vi "Mathematical_operations.vi"() -> ()   [LabVIEW 2019]
doc: "A vi which has the options to Add, Subtract, Multiply, Divide, Minimum and Maximum of two numbers namely A and B and to find the square and square root of A"
panel:
  in  "stop":bool
  in  "Enum":T1(ring)
  out "Result":dbl
  in  "B":dbl
  in  "A":dbl
  # "Mathematical Operations"
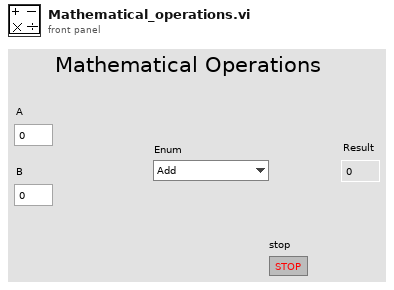
[diagram p1: front panel]
types:
  T1 = enum16{"Add", "Subtract", "Multiply", "Divide", "Square of A", "Square Root of A", "Average", "Minimum", "Maximum"}
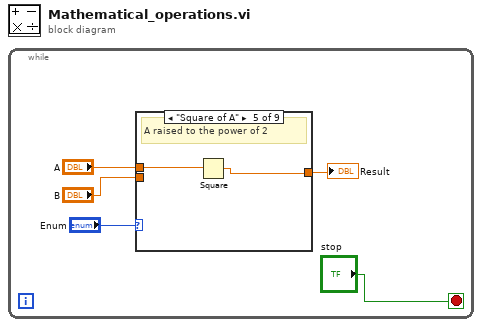
[diagram p0: block diagram]
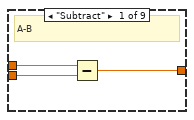
[diagram p2: hidden frame]
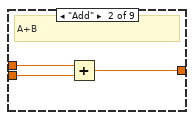
[diagram p3: hidden frame]
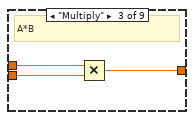
[diagram p4: hidden frame]
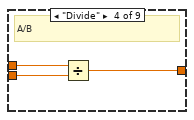
[diagram p5: hidden frame]
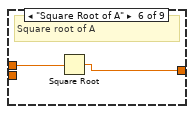
[diagram p6: hidden frame]
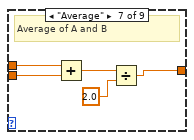
[diagram p7: hidden frame]
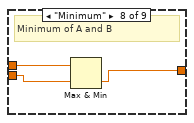
[diagram p8: hidden frame]
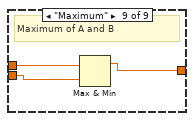
[diagram p9: hidden frame]
diagram:
  n1 = while {
    stop <- "stop" stop-if-true
    n2 = case shown="\"Square of A\"" "Enum" {
      tunnel: "A" -> [w8 w11 w14 w17 w19 w21 w26 w29 w32]
      tunnel: "B" -> [w7 w10 w13 w16 _ _ w25 w28 w31]
      tunnel: [w6 w9 w12 w15 w18 w20 w22 w27 w30] -> w2
      frame "Subtract" {
        # "A-B"
        n3 = Subtract(x=w8, y=w7) -> (x-y=w6:dbl)
      }
      frame "Add" {
        # "A+B"
        n4 = Add(x=w11, y=w10) -> (x+y=w9:dbl)
      }
      frame "Multiply" {
        # "A*B"
        n5 = Multiply(x=w14, y=w13) -> (x*y=w12:dbl)
      }
      frame "Divide" {
        # "A/B"
        n6 = Divide(x=w17, y=w16) -> (x/y=w15:dbl)
      }
      frame "Square of A" {
        # "A raised to the power of 2"
        n7 = Square(x=w19) -> (x^2=w18:dbl)
      }
      frame "Square Root of A" {
        # "Square root of A"
        n8 = Square Root(x=w21) -> (sqrt(x)=w20:dbl)
      }
      frame "Average" {
        # "Average of A and B"
        n9 = Add(x=w26, y=w25) -> (x+y=w24:dbl)
        n10 = Divide(x=w24, y=2.0) -> (x/y=w22:dbl)
      }
      frame "Minimum" {
        # "Minimum of A and B"
        n11 = Max & Min(x=w29, y=w28) -> (min(x,y)=w27:dbl)  [unwired: 1 out]
      }
      frame "Maximum" {
        # "Maximum of A and B"
        n12 = Max & Min(x=w32, y=w31) -> (max(x,y)=w30:dbl)  [unwired: 1 out]
      }
    }
    "Result" <- w2
  }
